vi "TTL_n_signals_gen.vi"() -> ()   [LabVIEW 2013]
uses:
  <vilib>/DAQmx/write.llb/DAQmx Write (Digital Bool 1Line 1Point).vi
  <vilib>/DAQmx/create/channels.llb/DAQmx Create Channel (DO-Digital Output).vi
  <vilib>/DAQmx/miscellaneous.llb/DAQmx Fill In Error Info.vi
panel:
  out ".not. x?":bool
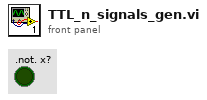
[diagram p1: front panel]
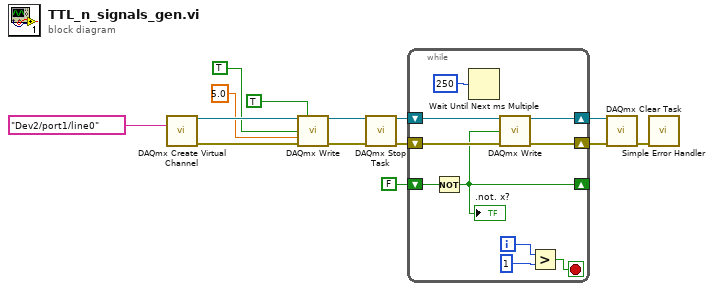
[diagram p0: block diagram]
diagram:
  n1 = call-poly <vilib>:"DAQmx Create Virtual Channel.vi"("lines"=tag "Dev2/port1/line0") -> ("task out"=w12:refnum<k21>, "error out"=w13:errorcluster)  [unwired: 13 in]
  n2 = call-poly <vilib>:"DAQmx Write.vi"("task/channels in"=w12, "auto start"=TRUE, "data"=TRUE, "timeout"=5.0, "error in"=w13) -> ("task out"=w7:refnum<k21>, "error out"=w11:errorcluster)  [unwired: 8 in, 1 out]
  n3 = call <vilib>:"DAQmx Stop Task.vi"("task/channels in"=w7, "error in"=w11) -> ("task out"=w6:refnum<k21>, "error out"=w8:errorcluster)  [unwired: 12 in]
  n4 = while {
    shift-right: [w21] -> w4
    shift-left: w8 -> [w24]
    shift-right: [w22] -> w5
    shift-left: w6 -> [w23]
    shift-right: [w18] -> _
    shift-left: FALSE -> [w19]
    i -> [w16]
    stop <- w17 stop-if-true
    n5 = Not(x=w19) -> (.not. x?=w18:bool)
    ".not. x?" <- w18
    n6 = Wait Until Next ms Multiple(millisecond multiple=u32 250) -> ()  [unwired: 1 out]
    n7 = call-poly <vilib>:"DAQmx Write.vi"("task/channels in"=w23, "data"=w18, "error in"=w24) -> ("task out"=w22:refnum<k21>, "error out"=w21:errorcluster)  [unwired: 10 in, 1 out]
    n8 = Greater?(x=w16, y=1) -> (0:w17:bool)
  }
  n9 = call <vilib>:"DAQmx Clear Task.vi"("task in"=w5, "error in"=w4) -> ("error out"=w3:errorcluster)  [unwired: 13 in]
  n10 = call <vilib>:"Simple Error Handler.vi"("error in (no error)"=w3) -> ()  [unwired: 4 in, 5 out]
